vi "check-up_adq.vi"(4 "JK(m/s)":dbl, 6 "JW(m/s)":dbl, 8 "P4(kPa)":dbl, 9 "P3(kPa)":dbl, 10 "P2(kPa)":dbl, 11 "P1(kPa)":dbl) -> (0 "OK 2 R":bool, 1 "OK 2 G":bool, 2 "OK RED":bool, 3 "OK G":bool)   [LabVIEW 2019]
panel:
  # "SE P1, P3 E P4 FOREM MENOR QUE 415,97 Pascal"
  # "SE P2 FOREM MENOR QUE 2074 Pascal"
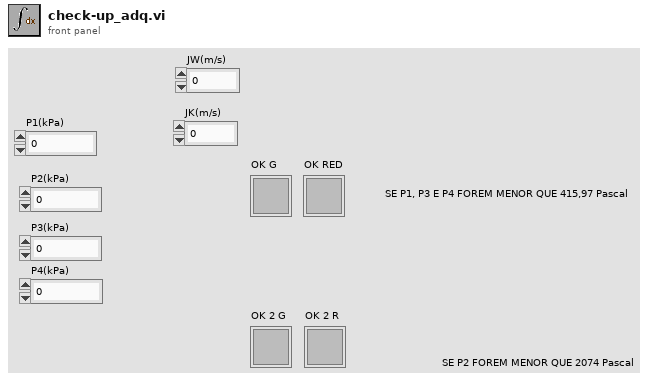
[diagram p1: front panel]
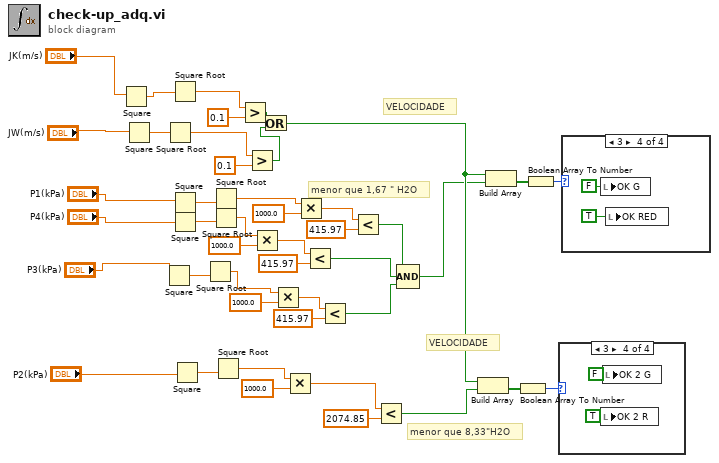
[diagram p0: block diagram]
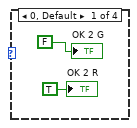
[diagram p2: hidden frame]
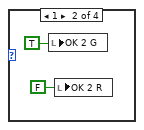
[diagram p3: hidden frame]
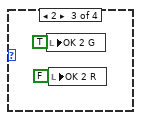
[diagram p4: hidden frame]
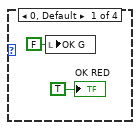
[diagram p5: hidden frame]
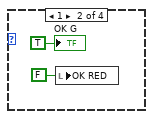
[diagram p6: hidden frame]
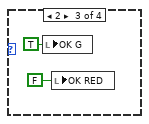
[diagram p7: hidden frame]
diagram:
  # "VELOCIDADE"
  # "menor que 8,33\"H2O"
  # "VELOCIDADE"
  # "menor que 1,67 \" H2O"
  n1 = Square(x="JK(m/s)") -> (x^2=w12:dbl)
  n2 = Square(x="JW(m/s)") -> (x^2=w13:dbl)
  n3 = Square(x="P3(kPa)") -> (x^2=w24:dbl)
  n4 = Square Root(x=w13) -> (sqrt(x)=w9:dbl)
  n5 = Square Root(x=w12) -> (sqrt(x)=w11:dbl)
  n6 = Square(x="P1(kPa)") -> (x^2=w44:dbl)
  n7 = Square(x="P4(kPa)") -> (x^2=w42:dbl)
  n8 = Square(x="P2(kPa)") -> (x^2=w43:dbl)
  n9 = Square Root(x=w24) -> (sqrt(x)=w23:dbl)
  n10 = Square Root(x=w44) -> (sqrt(x)=w37:dbl)
  n11 = Square Root(x=w42) -> (sqrt(x)=w36:dbl)
  n12 = Square Root(x=w43) -> (sqrt(x)=w39:dbl)
  n13 = Greater?(x=w11, y=0.1) -> (0:w14:bool)
  n14 = Greater?(x=w9, y=0.1) -> (0:w7:bool)
  n15 = Multiply(x=w36, y=1000.0) -> (x*y=w34:dbl)
  n16 = Or(x=w14, y=w7) -> (x .or. y?=w26:bool)
  n17 = Multiply(x=w23, y=1000.0) -> (x*y=w21:dbl)
  n18 = Multiply(x=w39, y=1000.0) -> (x*y=w31:dbl)
  n19 = Multiply(x=w37, y=1000.0) -> (x*y=w32:dbl)
  n20 = Less?(x=w34, y=415.97) -> (x < y?=w18:bool)
  n21 = Less?(x=w21, y=415.97) -> (x < y?=w19:bool)
  n22 = Less?(x=w32, y=415.97) -> (x < y?=w17:bool)
  n23 = Less?(x=w31, y=2074.85) -> (x < y?=w15:bool)
  n24 = Compound Arithmetic op=AND(w17, w18, w19) -> (w16:bool)
  n25 = Build Array(w26, w15) -> (w27:bool[])
  n26 = Build Array(w26, w16) -> (w29:bool[])
  n27 = Boolean Array To Number(Boolean array=w27) -> (number=w25:u32)
  n28 = Boolean Array To Number(Boolean array=w29) -> (number=w28:u32)
  n29 = case shown="3" w25 {
    frame 0, Default {
      "OK 2 G" <- FALSE ("OK")
      "OK 2 R" <- TRUE ("OK 2 R")
    }
    frame 1 {
      n30 = local write "OK 2 G"(TRUE ("OK")) -> ()
      n31 = local write "OK 2 R"(FALSE ("OK 2 R")) -> ()
    }
    frame 2 {
      n32 = local write "OK 2 G"(TRUE ("OK")) -> ()
      n33 = local write "OK 2 R"(FALSE ("OK")) -> ()
    }
    frame 3 {
      n34 = local write "OK 2 R"(TRUE ("OK")) -> ()
      n35 = local write "OK 2 G"(FALSE ("OK")) -> ()
    }
  }
  n36 = case shown="3" w28 {
    frame 0, Default {
      n37 = local write "OK G"(FALSE ("OK")) -> ()
      "OK RED" <- TRUE ("OK RED")
    }
    frame 1 {
      n38 = local write "OK RED"(FALSE ("OK RED")) -> ()
      "OK G" <- TRUE ("OK")
    }
    frame 2 {
      n39 = local write "OK G"(TRUE ("OK")) -> ()
      n40 = local write "OK RED"(FALSE ("OK RED")) -> ()
    }
    frame 3 {
      n41 = local write "OK G"(FALSE ("OK")) -> ()
      n42 = local write "OK RED"(TRUE ("OK RED")) -> ()
    }
  }
